vi "Transform RA-DEC to Alt-Az.vi"(4 "dec":dbl=-10.562198424995685 format="%#_11g", 6 "RA":dbl=205.47242696145108 format="%#_11g", 8 "LST [Deg]":ext=179.04613315298528775, 9 "Observer's Longitude":ext=105.2369444 format="%#_10g", 10 "Observer's Latitude (phi)":dbl=40.125, 11 "Greenwich Sideral Time":dbl=284.2830775973853 format="%#_12g") -> (2 "Az":dbl=148.26803884295992 format="%#_10g", 3 "Alt":dbl=33.71129618687101 format="%#_10g")   [LabVIEW 2015]
panel:
  out "H":ext=-26.42629380846579
  out "Local Hour Angle":dbl=-26.426293764065804
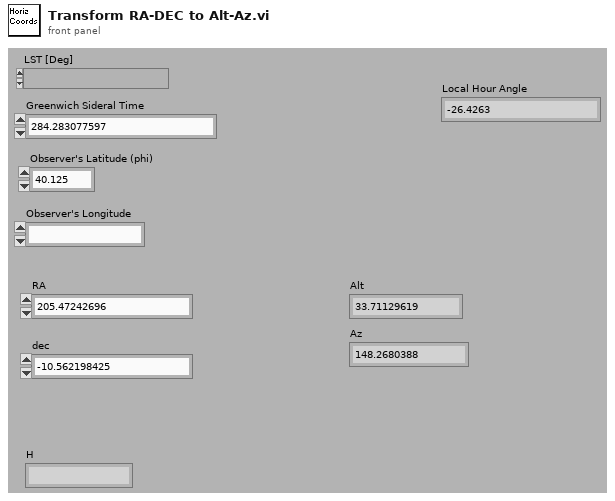
[diagram p1: front panel]
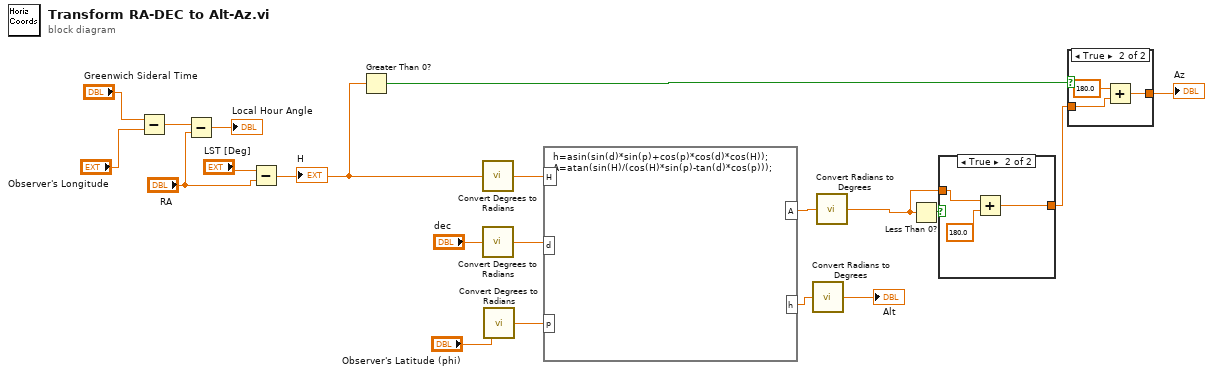
[diagram p0: block diagram]
diagram:
  n1 = Subtract(x="Greenwich Sideral Time", y="Observer's Longitude") -> (x-y=w18:ext)
  n2 = Subtract(x=w18, y="RA") -> (x-y=→"Local Hour Angle":ext)
  n3 = Subtract(x="LST [Deg]", y="RA") -> (x-y=w3:ext)
  "H" <- w3
  n4 = Greater Than 0?(x=w3) -> (x > 0?=w4:bool)
  n5 = call "Convert Degrees to Radians.vi"("degrees"=w3) -> ("radians"=w11:dbl)
  n6 = call "Convert Degrees to Radians.vi"("degrees"="dec") -> ("radians"=w10:dbl)
  n7 = call "Convert Degrees to Radians.vi"("degrees"="Observer's Latitude (phi)") -> ("radians"=w9:dbl)
  n8 = formula code="h=asin(sin(d)*sin(p)+cos(p)*cos(d)*cos(H));\nA=atan(sin(H)/(cos(H)*sin(p)-tan(d)*cos(p)));"("H"=w11, "d"=w10, "p"=w9) -> ("A"=w12:dbl, "h"=w7:dbl)
  n9 = call "Convert Radians to Degrees.vi"("radians"=w7) -> ("degrees"=→"Alt":dbl)
  n10 = call "Convert Radians to Degrees.vi"("radians"=w12) -> ("degrees"=w5:dbl)
  n11 = Less Than 0?(x=w5) -> (x < 0?=w6:bool)
  n12 = case shown="True" w6 {
    tunnel: w5 -> [w21 w23]
    tunnel: [w21 w22] -> w2
    frame False {
    }
    frame True {
      n13 = Add(x=w23, y=180.0) -> (x+y=w22:dbl)
    }
  }
  n14 = case shown="True" w4 {
    tunnel: w2 -> [w25 w27]
    tunnel: [w25 w26] -> w1
    frame False {
    }
    frame True {
      n15 = Add(x=180.0, y=w27) -> (x+y=w26:dbl)
    }
  }
  "Az" <- w1
